vi "finishUp.vi"(8 "error in (no error)":errorcluster, 11 "AtomChipHWC in":refnum<class "AtomChipHWC.lvclass">) -> (0 "error out":errorcluster, 3 "AtomChipHWC out":refnum<class "AtomChipHWC.lvclass">)   [LabVIEW 2011, in "Hardware.lvlib" / "HWControllers.lvlib" / "AtomChipHWC.lvclass"]
uses:
  AtomChipHWC.lvclass
  HWController.lvclass
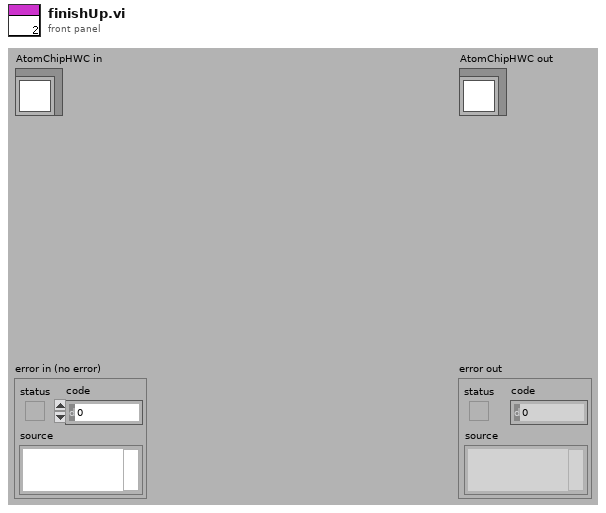
[diagram p1: front panel]
types:
  T1 = enum16{"Ready", "Compiling", "Configured", "Running", "Stopping", "Unresolved Error"}
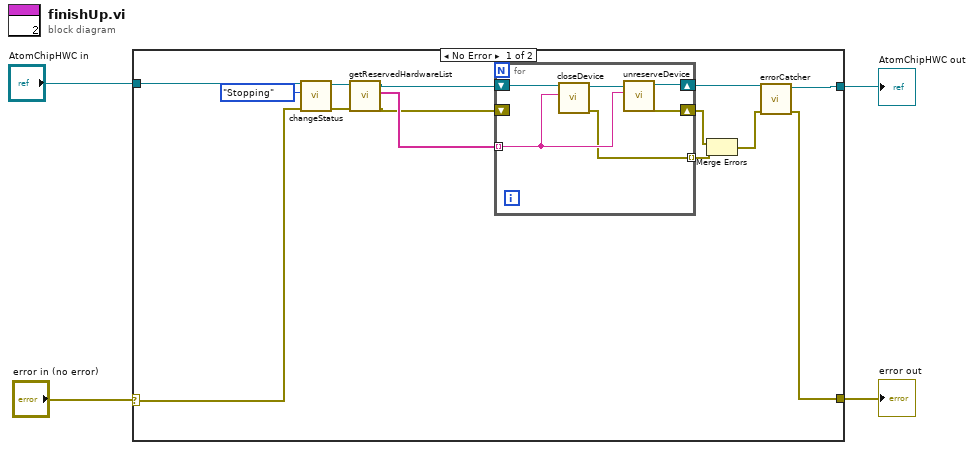
[diagram p0: block diagram]
diagram:
  n1 = case shown="No Error" "error in (no error)" {
    selector: "error in (no error)" -> [w14 w25]
    tunnel: "AtomChipHWC in" -> [w17 w26]
    tunnel: [w6 w26] -> w2
    tunnel: [w5 w25] -> w1
    frame No Error {
      n2 = call "changeStatus.vi"("error in (no error)"=w14, "status"=T1."Stopping", "HWController in"=w17) -> ("error out"=w15:errorcluster, "HWController out"=w16:refnum<class "AtomChipHWC.lvclass">)  [unwired: 7 in]
      n3 = call "getReservedHardwareList.vi"("error in (no error)"=w15, "HWController.lvclass in"=w16) -> ("error out"=w12:errorcluster, "reservedHardwareList"=w18:string[], "HWController.lvclass out"=w13:refnum<class "AtomChipHWC.lvclass">)  [unwired: 7 in]
      n4 = for {
        shift-right: [w22] -> w8
        shift-left: w13 -> [w24]
        shift-right: [w21] -> w10
        shift-left: w12 -> [_]
        tunnel: w18 -> [w20] mode=indexing
        tunnel: [w19] -> w11 mode=indexing
        n5 = call "closeDevice.vi"("deviceName"=w20, "AtomChipHWC in"=w24) -> ("error out"=w19:errorcluster, "AtomChipHWC out"=w23:refnum<class "AtomChipHWC.lvclass">)  [unwired: 8 in]
        n6 = call "unreserveDevice.vi"("deviceName"=w20, "HWController.lvclass in"=w23) -> ("error out"=w21:errorcluster, "HWController.lvclass out"=w22:refnum<class "AtomChipHWC.lvclass">)  [unwired: 8 in]
      }
      n7 = Merge Errors(w10, w11) -> (w7:errorcluster)
      n8 = call-dynamic "errorCatcher.vi"("error in (no error)"=w7, "HWController in"=w8) -> ("error out"=w5:errorcluster, "HWController out"=w6:refnum<class "AtomChipHWC.lvclass">)  [unwired: 8 in]
    }
    frame Error {
    }
  }
  "error out" <- w1
  "AtomChipHWC out" <- w2
